vi "PCBdummySiCenterFinder_old.vi"() -> ()   [LabVIEW 2019]
uses:
  <vilib>/userDefined/High Color/IMAQdx.ctl
  Other Models/2010/Motion/AbortSingle.vi
panel:
  in  "VisibilityInCamera":enum16{"JoyStick", "ClickToMove", "AllVisible"}(ring)
  out "UsedCoordinates":string
  in  "AdjustCamera":T1={"+Y"=FALSE, "-Z"=FALSE, "Done"=FALSE, "+Z"=FALSE, "-Y"=FALSE, "-X"=FALSE, "+X"=FALSE, "MoveXYBy(mm)"=0.25, "MoveZBy(mm)"=0.1} {"MoveZBy(mm)" format="%#_13g"}
  in  "StopJoyStick":bool
  out "CameraGcode":string
  out "Image":T2(plugin-control)
  out "Deviation":dbl
  out "Output XYZU":string
  in  "PCBCorners":path=path "C:/Users/TTUHEP/Documents/LabVIEW/GantryPrograms/Configs/PCB1_4PointsA1.txt"
  in  "SiNoPatternCorners":path=path "C:/Users/TTUHEP/Documents/LabVIEW/GantryPrograms/Configs/SiDummy1Corners.txt"
  in  "Component":enum16{"SiNoPattern", "PCB"}(ring)
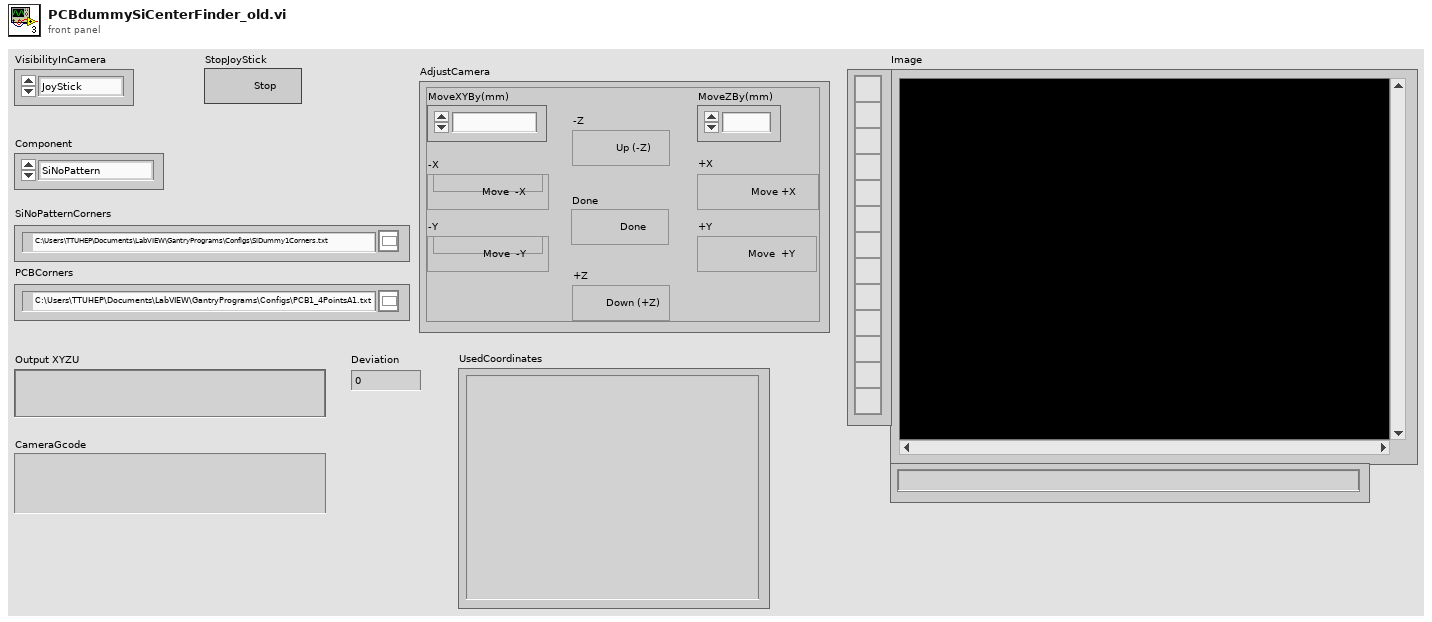
[diagram p1: front panel]
types:
  T1 = cluster{"+Y":bool, "-Z":bool, "Done":bool, "+Z":bool, "-Y":bool, "-X":bool, "+X":bool, "MoveXYBy(mm)":dbl, "MoveZBy(mm)":dbl}
  T2 = typedef "IMAQ Image.ctl" = refnum<image>
  T3 = typedef "IMAQdx.ctl" = refnum<k21>
  T4 = typedef "IMAQ Point" = cluster{"X":sgl, "Y":sgl}
  T5 = enum16{"Left Button", "Center Button", "Right Button", "Window Close"}
  T6 = enum16{"open", "replace", "create", "open or create", "replace or create", "replace or create with confirmation"}
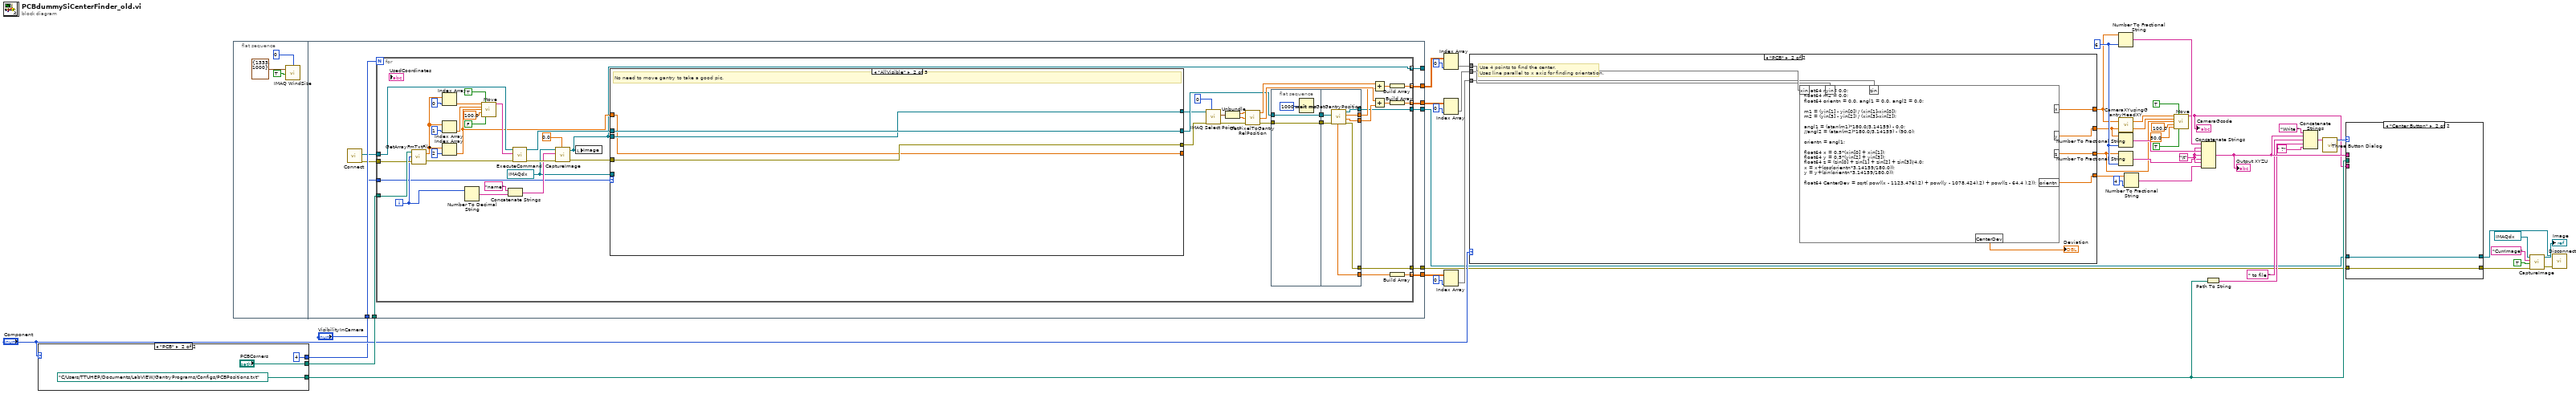
[diagram p0: block diagram]
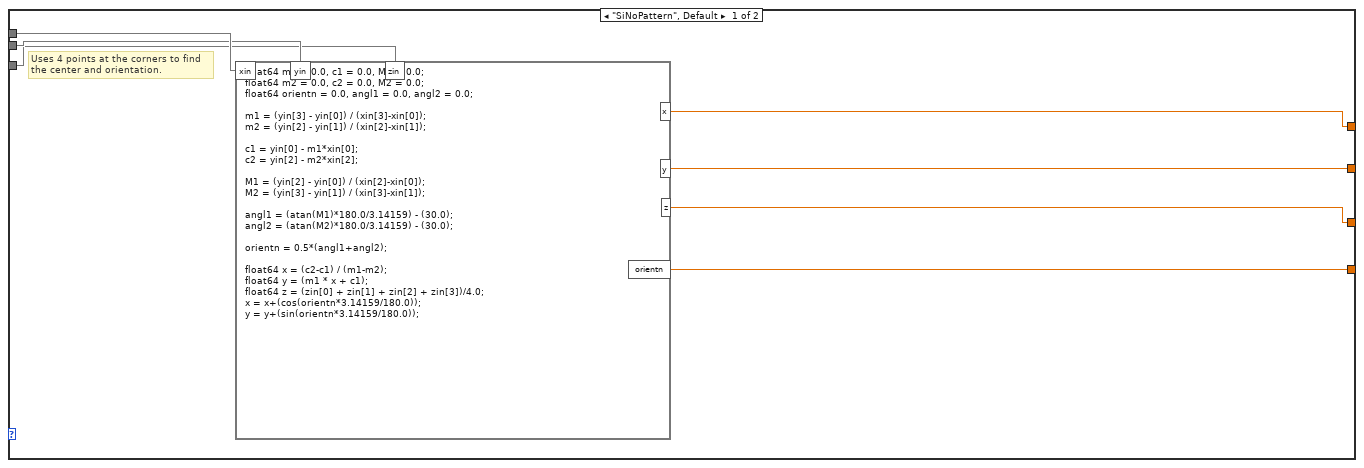
[diagram p2: hidden frame]
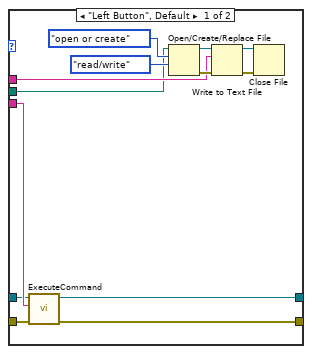
[diagram p3: hidden frame]
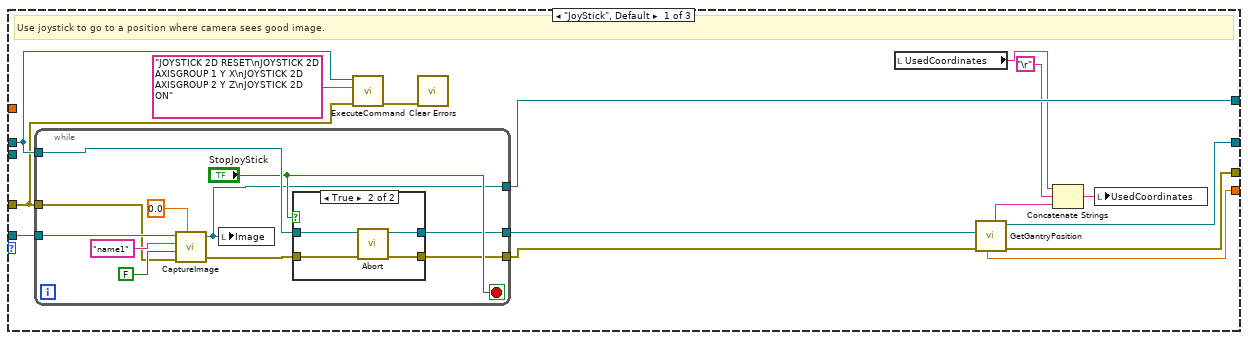
[diagram p4: hidden frame]
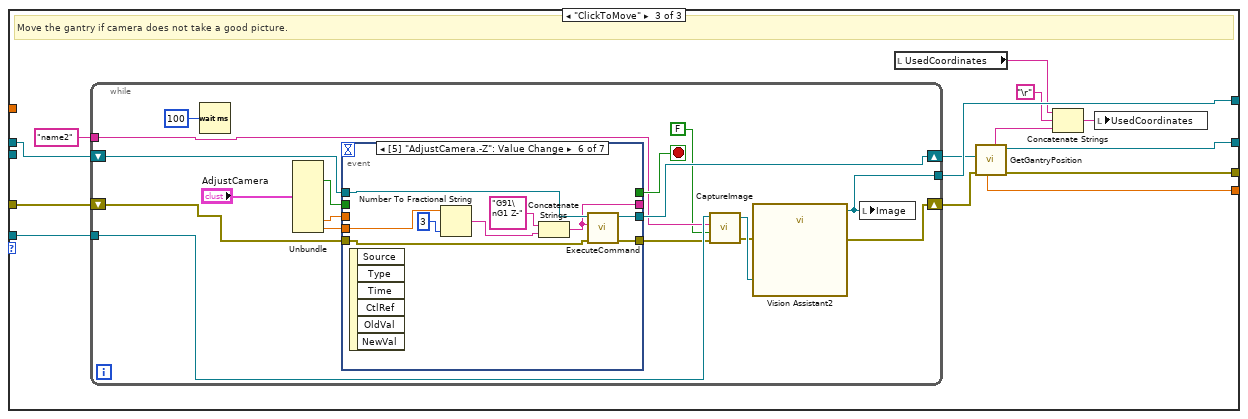
[diagram p6: hidden frame]
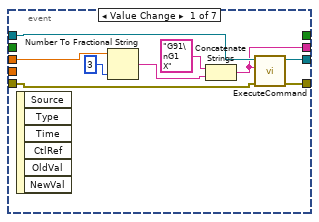
[diagram p7: hidden frame]
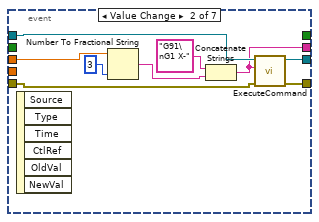
[diagram p8: hidden frame]
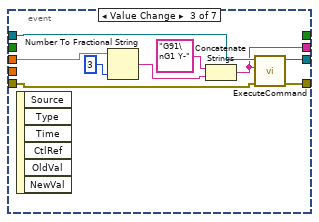
[diagram p9: hidden frame]
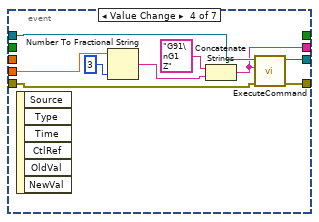
[diagram p10: hidden frame]
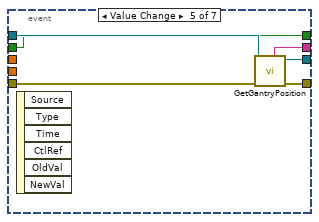
[diagram p11: hidden frame]
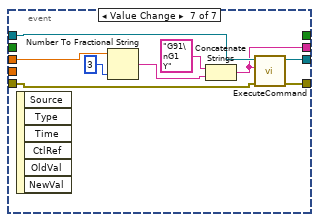
[diagram p12: hidden frame]
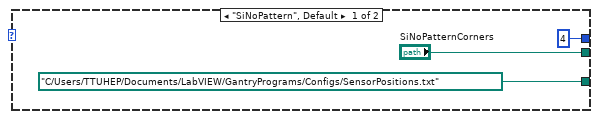
[diagram p13: hidden frame]
diagram:
  w45 = "\t"
  w42 = i16 6 ("width (-)")
  n1 = case shown="\"PCB\"" "Component" {
    tunnel: ["SiNoPatternCorners" "PCBCorners"] -> w48
    tunnel: [path "C:/Users/TTUHEP/Documents/LabVIEW/GantryPrograms/Configs/SensorPositions.txt" ("OutFile") path "C:/Users/TTUHEP/Documents/LabVIEW/GantryPrograms/Configs/PCBPositions.txt" ("OutFile")] -> w33
    tunnel: [4 4] -> w9
    frame "SiNoPattern", Default {
    }
    frame "PCB" {
    }
  }
  n2 = flat-sequence {
    tunnel: w9 -> [w68]
    tunnel: w48 -> [w67]
    tunnel: [w66] -> w7
    tunnel: [w65] -> w5
    tunnel: [w62] -> _
    tunnel: [w61] -> w31
    tunnel: [w60] -> w27
    tunnel: [w59] -> w29
    tunnel: "VisibilityInCamera" -> [w58]
    frame #0 {
      n3 = call "IMAQ WindSize"("Scrollbars? (N)"=TRUE, "Width & Height"=cluster{"Width":i32, "Height":i32} {"Width"=1333, "Height"=1000}, "Window Number"=0) -> ()  [unwired: 3 in, 3 out]
    }
    frame #1 {
      n4 = call "Connect.vi"() -> ("error out"=w64:errorcluster, "controller"=w63:refnum<k24>)  [unwired: 10 in]
      n5 = for {
        N: w68 -> [_]
        tunnel: w67 -> [w113]
        tunnel: w63 -> [w106]
        tunnel: w64 -> [w105]
        tunnel: [w85] -> w66
        tunnel: [w82] -> w65
        tunnel: [w72] -> w62 mode=indexing
        tunnel: [w99] -> w61 mode=indexing
        tunnel: [w94] -> w60 mode=indexing
        tunnel: [w93] -> w59 mode=indexing
        tunnel: w58 -> [w70]
        i -> [w103]
        w77 = T3 "cam1" ("Camera")
        n6 = call "GetArrayFmTxtFile.vi"("error in"=w105, "LineNo."=w103, "TextFile"=w113) -> ("error out"=w104:errorcluster, "Array"=w114:dbl[])
        n7 = Index Array(array=w114, index=0) -> (element=w91:dbl)
        n8 = Index Array(array=w114, index=1) -> (element=w89:dbl)
        n9 = Index Array(array=w114, index=2) -> (element=w73:dbl)
        n10 = Number To Decimal String(number=w103) -> (decimal integer string=w102:string)  [unwired: 1 in]
        n11 = call "Move.vi"("X"=w91, "Absolute"=TRUE, "Y"=w89, "Z"=w73, "SpeedXY (mm/s)"=100.0, "Move Z first"=FALSE) -> ("Position Gcode"=w107:string)  [unwired: 9 in]
        n12 = Concatenate Strings("name" ("string"), w102) -> (w100:string)
        n13 = call "ExecuteCommand.vi"("error in (no error)"=w104, "Command Code"=w107, "controller in"=w106) -> ("error out"=w109:errorcluster, "controller out"=w75:refnum<k24>)  [unwired: 6 in, 1 out]
        n14 = call "CaptureImage.vi"("Camera"=w77, "Rotate (degrees)"=sgl 0.0, "ImageName"=w100, "error in (no error)"=w109) -> ("Image"=w72:T2, "error out"=w76:errorcluster)  [unwired: 3 in]
        n15 = local write "Image"(w72) -> ()
        n16 = case shown="\"AllVisible\"" w70 {
          tunnel: w77 -> [w131 _ w166]
          tunnel: w75 -> [w129 w152 w165]
          tunnel: w76 -> [w127 w153 w164]
          tunnel: [w130 w151 w163] -> w71
          tunnel: [w125 w152 w156] -> w74
          tunnel: [w123 w153 w154] -> w69
          tunnel: w72 -> [_ w151 _]
          tunnel: [w118 w150 w155] -> _
          tunnel: w73 -> [_ w150 _]
          frame "JoyStick", Default {
            # "Use joystick to go to a position where camera sees good image."
            n17 = while {
              tunnel: w131 -> [w142]
              tunnel: [w133] -> w130
              tunnel: w129 -> [w139]
              tunnel: [w136] -> w124
              tunnel: [w135] -> w126
              tunnel: w127 -> [w134]
              stop <- "StopJoyStick" stop-if-true
              n18 = call "CaptureImage.vi"("Camera"=w142, "Rotate (degrees)"=sgl 0.0, "ImageName"="name1", "Draw50MicroCircleAtCenter"=FALSE, "error in (no error)"=w134) -> ("Image"=w133:T2, "error out"=w137:errorcluster)  [unwired: 2 in]
              n19 = local write "Image"(w133) -> ()
              n20 = case shown="True" "StopJoyStick" {
                tunnel: w139 -> [w145 w149]
                tunnel: w137 -> [w144 w148]
                tunnel: [w144 w147] -> w136
                tunnel: [w145 w146] -> w135
                frame False {
                }
                frame True {
                  n21 = call-poly "Abort.vi"("error in (no error)"=w148, "controller in"=w149) -> ("error out"=w147:errorcluster, "controller out"=w146:refnum<k24>)  [unwired: 8 in]
                }
              }
            }
            n22 = call "ExecuteCommand.vi"("error in (no error)"=w127, "Command Code"="JOYSTICK 2D RESET\nJOYSTICK 2D AXISGROUP 1 Y X\nJOYSTICK 2D AXISGROUP 2 Y Z\nJOYSTICK 2D ON", "controller in"=w129) -> ("error out"=w128:errorcluster)  [unwired: 6 in, 2 out]
            n23 = call <vilib>:"Clear Errors.vi"("error in (no error)"=w128) -> ()  [unwired: 5 in, 2 out]
            n24 = local read "UsedCoordinates"() -> (w121:string)
            n25 = call "GetGantryPosition.vi"("error in (no error)"=w124, "Controller In"=w126) -> ("error out"=w123:errorcluster, "controller out"=w125:refnum<k24>, "Position_XYZ"=w119:string, "Position Z"=w118:dbl)  [unwired: 3 in, 3 out]
            n26 = Concatenate Strings(w121, "\r", w119) -> (w122:string)
            n27 = local write "UsedCoordinates"(w122) -> ()
          }
          frame "AllVisible" {
            # "No need to move gantry to take a good pic."
          }
          frame "ClickToMove" {
            # "Move the gantry if camera does not take a good picture."
            n28 = while {
              shift-right: [w176] -> w158
              shift-left: w164 -> [w184]
              shift-right: [w182] -> w157
              shift-left: w165 -> [w183]
              tunnel: "name2" ("ImageName") -> [w178]
              tunnel: w166 -> [w179]
              tunnel: [w168] -> w163
              stop <- w181 stop-if-true
              n29 = Wait (ms)(milliseconds to wait=u32 100) -> ()  [unwired: 1 out]
              n30 = Unbundle("AdjustCamera") -> ("Done"=w172:bool, "MoveXYBy(mm)"=w170:dbl, "MoveZBy(mm)"=w171:dbl)  [unwired: 6 out]
              n31 = event shown="[5] \"AdjustCamera.-Z\": Value Change" {
                selector: _ -> [_ _ _ _ _ _ _]
                dyn-events: _ -> [_ _ _ _ _ _ _]
                timeout: _ -> [_ _ _ _ _ _ _]
                tunnel: w170 -> [w190 w194 w203 _ _ _ w236]
                tunnel: w184 -> [w189 w198 w207 w216 w225 w231 w240]
                tunnel: [w188 w197 w206 w213 w222 w230 w239] -> w177
                tunnel: w183 -> [w187 w199 w208 w217 w226 w232 w241]
                tunnel: [w186 w196 w205 w214 w224 w229 w238] -> w182
                tunnel: [w185 w195 w204 w215 w223 w228 w237] -> _
                tunnel: [_ _ _ _ w221 _ _] -> w181
                tunnel: w171 -> [_ _ _ w212 _ w227 _]
                tunnel: w172 -> [_ _ _ _ w221 _ _]
                event "AdjustCamera.+X": Value Change {
                  n32 = event-data() -> ()  [unwired: 1 in, 6 out]
                  n33 = Number To Fractional String(number=w190, precision (6)=3) -> (F-format string=w193:string)  [unwired: 2 in]
                  n34 = Concatenate Strings("G91\nG1 X", w193) -> (w185:string)
                  n35 = call "ExecuteCommand.vi"("error in (no error)"=w189, "Command Code"=w185, "controller in"=w187) -> ("error out"=w188:errorcluster, "controller out"=w186:refnum<k24>)  [unwired: 6 in, 1 out]
                }
                event "AdjustCamera.-X": Value Change {
                  n36 = event-data() -> ()  [unwired: 1 in, 6 out]
                  n37 = Number To Fractional String(number=w194, precision (6)=3) -> (F-format string=w202:string)  [unwired: 2 in]
                  n38 = Concatenate Strings("G91\nG1 X-", w202) -> (w195:string)
                  n39 = call "ExecuteCommand.vi"("error in (no error)"=w198, "Command Code"=w195, "controller in"=w199) -> ("error out"=w197:errorcluster, "controller out"=w196:refnum<k24>)  [unwired: 6 in, 1 out]
                }
                event "AdjustCamera.-Y": Value Change {
                  n40 = event-data() -> ()  [unwired: 1 in, 6 out]
                  n41 = Number To Fractional String(number=w203, precision (6)=3) -> (F-format string=w211:string)  [unwired: 2 in]
                  n42 = Concatenate Strings("G91\nG1 Y-", w211) -> (w204:string)
                  n43 = call "ExecuteCommand.vi"("error in (no error)"=w207, "Command Code"=w204, "controller in"=w208) -> ("error out"=w206:errorcluster, "controller out"=w205:refnum<k24>)  [unwired: 6 in, 1 out]
                }
                event "AdjustCamera.+Z": Value Change {
                  n44 = event-data() -> ()  [unwired: 1 in, 6 out]
                  n45 = Number To Fractional String(number=w212, precision (6)=3) -> (F-format string=w220:string)  [unwired: 2 in]
                  n46 = Concatenate Strings("G91\nG1 Z", w220) -> (w215:string)
                  n47 = call "ExecuteCommand.vi"("error in (no error)"=w216, "Command Code"=w215, "controller in"=w217) -> ("error out"=w213:errorcluster, "controller out"=w214:refnum<k24>)  [unwired: 6 in, 1 out]
                }
                event "AdjustCamera.Done": Value Change {
                  n48 = event-data() -> ()  [unwired: 1 in, 6 out]
                  n49 = call "GetGantryPosition.vi"("error in (no error)"=w225, "Controller In"=w226) -> ("error out"=w222:errorcluster, "controller out"=w224:refnum<k24>, "Position_XYZ"=w223:string)  [unwired: 3 in, 4 out]
                }
                event "AdjustCamera.-Z": Value Change {
                  n50 = event-data() -> ()  [unwired: 1 in, 6 out]
                  n51 = Number To Fractional String(number=w227, precision (6)=3) -> (F-format string=w235:string)  [unwired: 2 in]
                  n52 = Concatenate Strings("G91\nG1 Z-", w235) -> (w228:string)
                  n53 = call "ExecuteCommand.vi"("error in (no error)"=w231, "Command Code"=w228, "controller in"=w232) -> ("error out"=w230:errorcluster, "controller out"=w229:refnum<k24>)  [unwired: 6 in, 1 out]
                }
                event "AdjustCamera.+Y": Value Change {
                  n54 = event-data() -> ()  [unwired: 1 in, 6 out]
                  n55 = Number To Fractional String(number=w236, precision (6)=3) -> (F-format string=w244:string)  [unwired: 2 in]
                  n56 = Concatenate Strings("G91\nG1 Y", w244) -> (w237:string)
                  n57 = call "ExecuteCommand.vi"("error in (no error)"=w240, "Command Code"=w237, "controller in"=w241) -> ("error out"=w239:errorcluster, "controller out"=w238:refnum<k24>)  [unwired: 6 in, 1 out]
                }
              }
              n58 = call "CaptureImage.vi"("Camera"=w179, "ImageName"=w178, "Draw50MicroCircleAtCenter"=FALSE, "error in (no error)"=w177) -> ("Image"=w175:T2, "error out"=w174:errorcluster)  [unwired: 3 in]
              n59 = call "Vision Assistant2"("Image In"=w175, "error in"=w174) -> ("Image Out"=w168:T2, "error out"=w176:errorcluster)  [unwired: 24 in]
              n60 = local write "Image"(w168) -> ()
            }
            n61 = local read "UsedCoordinates"() -> (w161:string)
            n62 = call "GetGantryPosition.vi"("error in (no error)"=w158, "Controller In"=w157) -> ("error out"=w154:errorcluster, "controller out"=w156:refnum<k24>, "Position_XYZ"=w159:string, "Position Z"=w155:dbl)  [unwired: 3 in, 3 out]
            n63 = Concatenate Strings(w161, "\r", w159) -> (w162:string)
            n64 = local write "UsedCoordinates"(w162) -> ()
          }
        }
        n65 = call "IMAQ Select Point"("Window Number (0...15)"=0, "error in (no error)"=w69, "Image In"=w71) -> ("error out"=w95:errorcluster, "Point"=w98:T4)  [unwired: 5 in, 2 out]
        n66 = Unbundle(w98) -> ("X"=w97:sgl, "Y"=w96:sgl)
        n67 = call "GetPixelToGantryRelPosition.vi"("error in (no error)"=w95, "PixelY"=w96, "PixelX"=w97) -> ("error out"=w80:errorcluster, "YmmRelGH"=w88:dbl, "XmmRelGH"=w92:dbl)
        n68 = flat-sequence {
          tunnel: w80 -> [w246]
          tunnel: [w246] -> w79
          tunnel: w74 -> [w245]
          tunnel: [w245] -> w78
          tunnel: [w254] -> w85
          tunnel: [w253] -> w84
          tunnel: [w252] -> w83
          tunnel: [w251] -> w82
          tunnel: [w250] -> w81
          tunnel: w79 -> [w249]
          tunnel: w78 -> [w248]
          frame #0 {
            n69 = Wait (ms)(milliseconds to wait=u32 1000) -> ()  [unwired: 1 out]
          }
          frame #1 {
            n70 = call "GetGantryPosition.vi"("error in (no error)"=w249, "Controller In"=w248) -> ("error out"=w254:errorcluster, "Position Y"=w253:dbl, "Position X"=w252:dbl, "controller out"=w251:refnum<k24>, "Position Z"=w250:dbl)  [unwired: 3 in, 2 out]
          }
        }
        n71 = Add(x=w92, y=w83) -> (x+y=w90:dbl)
        n72 = Add(x=w88, y=w84) -> (x+y=w87:dbl)
        n73 = Build Array(w90) -> (w93:dbl[])
        n74 = Build Array(w87) -> (w94:dbl[])
        n75 = Build Array(w81) -> (w99:dbl[])
      }
    }
  }
  n76 = Index Array(array=w29, index (col)=0 ("disabled index (col)")) -> (element=w26:dbl[])  [unwired: 1 in]
  n77 = Index Array(array=w27, index (col)=0 ("disabled index (col)")) -> (element=w25:dbl[])  [unwired: 1 in]
  n78 = Index Array(array=w31, index (col)=0 ("disabled index (col)")) -> (element=w24:dbl[])  [unwired: 1 in]
  n79 = case shown="\"PCB\"" "Component" {
    tunnel: w26 -> [w261 w269]
    tunnel: w25 -> [w260 w268]
    tunnel: w24 -> [w259 w267]
    tunnel: [w258 w266] -> w23
    tunnel: [w257 w265] -> w14
    tunnel: [w256 w264] -> w13
    tunnel: [w255 w263] -> w10
    frame "SiNoPattern", Default {
      # "Uses 4 points at the corners to find\nthe center and orientation."
      n80 = formula code="float64 m1 = 0.0, c1 = 0.0, M1 = 0.0;\nfloat64 m2 = 0.0, c2 = 0.0, M2 = 0.0;\nfloat64 orientn = 0.0, angl1 = 0.0, angl2 = 0.0;\n\nm1 = (yin[3] - yin[0]) / (xin[3]-xin[0]);\nm2 = (yin[2] - yin[1]) / (xin[2]-xin[1]);\n\nc1 = yin[0] - m1*xin[0];\nc2 = yin[2] - m2*xin[2];\n\nM1 = (yin[2] - yin[0]) / (xin[2]-xin[0]);\nM2 = (yin[3] - yin[1]) / (xin[3]-xin[1]);\n\nangl1 = (atan(M1)*180.0/3.14159) - (30.0);\nangl2 = (atan(M2)*180.0/3.14159) - (30.0);\n\norientn = 0.5*(angl1+angl2);\n\nfloat64 x = (c2-c1) / (m1-m2);\nfloat64 y = (m1 * x + c1);\nfloat64 z = (zin[0] + zin[1] + zin[2] + zin[3])/4.0;\nx = x+(cos(orientn*3.14159/180.0));\ny = y+(sin(orientn*3.14159/180.0));"("xin"=w261, "yin"=w260, "zin"=w259) -> ("orientn"=w258:dbl, "x"=w257:dbl, "y"=w256:dbl, "z"=w255:dbl)
    }
    frame "PCB" {
      # "Use 4 points to find the center.\nUses line parallel to x axis for finding orientation."
      n81 = formula code="float64 m1 = 0.0;\nfloat64 m2 = 0.0;\nfloat64 orientn = 0.0, angl1 = 0.0, angl2 = 0.0;\n\nm1 = (yin[1] - yin[0]) / (xin[1]-xin[0]);\nm2 = (yin[3] - yin[2]) / (xin[3]-xin[2]);\n\nangl1 = (atan(m1)*180.0/3.14159) - 0.0;\n//angl2 = (atan(m2)*180.0/3.14159) - (90.0);\n\norientn = angl1;\n\nfloat64 x = 0.5*(xin[0] + xin[1]);\nfloat64 y = 0.5*(yin[2] + yin[3]);\nfloat64 z = (zin[0] + zin[1] + zin[2] + zin[3])/4.0;\nx = x+(cos(orientn*3.14159/180.0));\ny = y+(sin(orientn*3.14159/180.0));\n\nfloat64 CenterDev = sqrt( pow((x - 1123.476),2) + pow((y - 1078.424),2) + pow((z - 64.4 ),2));"("xin"=w269, "yin"=w268, "zin"=w267) -> ("orientn"=w266:dbl, "x"=w265:dbl, "y"=w264:dbl, "z"=w263:dbl, "CenterDev"=→"Deviation":dbl)
    }
  }
  n82 = Number To Fractional String(number=w14, precision (6)=w42) -> (F-format string=w47:string)  [unwired: 2 in]
  n83 = call "CameraXYusingGantryHeadXY.vi"("GantryY"=w13, "GantryX"=w14) -> ("CamY"=w11:dbl, "CamX"=w12:dbl)
  n84 = Number To Fractional String(number=w13, precision (6)=w42) -> (F-format string=w46:string)  [unwired: 2 in]
  n85 = Number To Fractional String(number=w10, precision (6)=w42) -> (F-format string=w41:string)  [unwired: 2 in]
  n86 = Number To Fractional String(number=w23, precision (6)=i16 4 ("width (-)")) -> (F-format string=w43:string)  [unwired: 2 in]
  n87 = call "Move.vi"("X"=w12, "Absolute"=TRUE, "Y"=w11, "Z"=w10, "SpeedXY (mm/s)"=100.0, "SpeedZ (mm/s)"=50.0, "Move Z first"=TRUE) -> ("Position Gcode"=w6:string)  [unwired: 8 in]
  "CameraGcode" <- w6
  n88 = Concatenate Strings(w47, w45, w46, w45, w41, w45, w43) -> (w39:string)
  "Output XYZU" <- w39
  n89 = Path To String(path=w33) -> (string=w37:string)
  n90 = Concatenate Strings("Write ", w39, " to file ", w37, " ?" ("string")) -> (w35:string)
  n91 = call <vilib>:"Three Button Dialog.vi"("message"=w35) -> ("Which Button?"=w34:T5)  [unwired: 10 in]
  n92 = case shown="\"Center Button\"" w34 {
    tunnel: w39 -> [w276 _]
    tunnel: w33 -> [w275 _]
    tunnel: w7 -> [w274 w284]
    tunnel: w6 -> [w273 _]
    tunnel: w5 -> [w272 w283]
    tunnel: [w271 w284] -> w4
    tunnel: [w270 w283] -> w3
    frame "Left Button", Default {
      n93 = call "ExecuteCommand.vi"("error in (no error)"=w274, "Command Code"=w273, "controller in"=w272) -> ("error out"=w271:errorcluster, "controller out"=w270:refnum<k24>)  [unwired: 6 in, 1 out]
      n94 = Open/Create/Replace File(file path (use dialog)=w275, operation (0:open)=T6."open or create", access (0:read/write)=enum16{"read/write", "read-only", "write-only"}."read/write") -> (refnum out=w282:refnum<file>, error out=w279:errorcluster)  [unwired: 3 in, 1 out]
      n95 = Write to Text File(file (use dialog)=w282, text=w276, error in=w279) -> (refnum out=w277:refnum<file>, error out=w278:errorcluster)  [unwired: 1 in, 1 out]
      n96 = Close File(refnum=w277, error in=w278) -> ()  [unwired: 2 out]
    }
    frame "Center Button" {
    }
  }
  n97 = call "CaptureImage.vi"("Camera"=T3 "cam1", "ImageName"="CurrImage", "Draw50MicroCircleAtCenter"=TRUE, "error in (no error)"=w4) -> ("Image"=→"Image":T2, "error out"=w17:errorcluster)  [unwired: 3 in]
  n98 = call "Disconnect.vi"("error in (no error)"=w17, "controller"=w3) -> ()  [unwired: 9 in, 1 out]
